vi "macro_DiffDrv_Sim_Execute.vi"() -> ()   [LabVIEW 2019, in "Trajectory_Library.lvlib"]
uses:
  Trajectory_Library.lvlib
  Enum/DCMOTOR_TYPES_ENUM.ctl
  Enum/DIFF_DRIVE_ToughBoxMini_GearChoice_ENUM.ctl
  Enum/DIFF_DRIVE_TRAIN_SIM_STATE_ENUM.ctl
  BatterySim_CalculateLoadedBatteryVoltage.vi
panel:
  in  "Right Motor Dmd (CO)":dbl
  in  "Left Motor Dmd (CO)":dbl
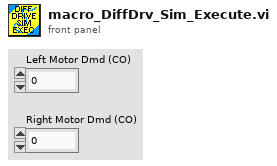
[diagram p1: front panel]
types:
  T1 = typedef "Trajectory_Library.lvlib/DIFF_DRIVE_TRAIN_SIM_STATE_ENUM.ctl" = enum16{"X_POS", "Y_POS", "HEADING", "LEFT_VEL", "RIGHT_VEL", "LEFT_DIST", "RIGHT_DIST"}
  T2 = typedef "Trajectory_Library.lvlib/DIFF_DRIVE_ToughBoxMini_GearChoice_ENUM.ctl" = enum16{"Ratio_12_75", "Ratio_10_71", "Ratio_8_45", "Ratio_7_31", "Ratio_5_95"}
  T3 = typedef "Trajectory_Library.lvlib/DCMOTOR_TYPES_ENUM.ctl" = enum16{"CIM", "AndyMark 9015", "Andy Mark RS 775 125", "Bag", "BaneBots RS 550", "BaneBots RS 775", "Falcon 500", "Mini CIM", "NEO", "NEO 550", "Romi BuiltIn", "Vex 775 Pro", "Snow Blower AM 2235A", "Bosch Seat AM 3493"}
  T4 = typedef "Trajectory_Library.lvlib/DIFF_DRIVE_SIM_SIMULATION_PARAMS.ctl" = cluster{"X Pos Meas Std Dev M":dbl, "Y Pos Meas Std Dev M":dbl, "Heading Meas Std Dev Rad":dbl, "Left Vel Meas Std Dev M/S":dbl, "Right Vel Meas Std Dev M/S":dbl, "Left Pos Meas Std Dev M":dbl, "Right Pos Meas Std Dev M":dbl}
  T5 = typedef "Trajectory_Library.lvlib/DIFF_DRIVE_SIM_MODEL_PARAMS.CTL" = cluster{"TracWidth_M":dbl, "WheelRadius_M":dbl, "Gearing":dbl, "Mass kg":dbl, "MOI kgm2":dbl, "DCMOTOR_TYPES":T3, "Num Motors":i32}
  T6 = typedef "Trajectory_Library.lvlib/DIFF_DRIVE_TRAIN_SIM.ctl" = cluster{"m_Plant":T7, "m_X":T8, "m_Y":T8, "m_U":T8, "MeasureStdDev":T8, "m_Motor":T9, "m_OriginalGearing":dbl, "m_CurrentGearing":dbl, "m_WheelRadius_M":dbl, "m_RB":dbl}
  T7 = typedef "Trajectory_Library.lvlib/LINEAR_SYSTEM.ctl" = cluster{"m_A":T8, "m_B":T8, "m_C":T8, "m_D":T8, "States":i32, "Inputs":i32, "Outputs":i32}
  T8 = typedef "NI_Matrix.lvlib/RealMatrix.ctl" = dbl[][]
  T9 = typedef "Trajectory_Library.lvlib/DCMOTOR.CTL" = cluster{"nominalVoltage_Volts":dbl, "StallTorque_NM":dbl, "StallCurrent_Amps":dbl, "FreeCurrent_Amps":dbl, "FreeSpeed_RadPerSec":dbl, "R_Ohms":dbl, "KvINV_RadPerSecPerVolt":dbl, "Kt_NMPerAmp":dbl, "L_H":dbl, "Jr_KgM2":dbl}
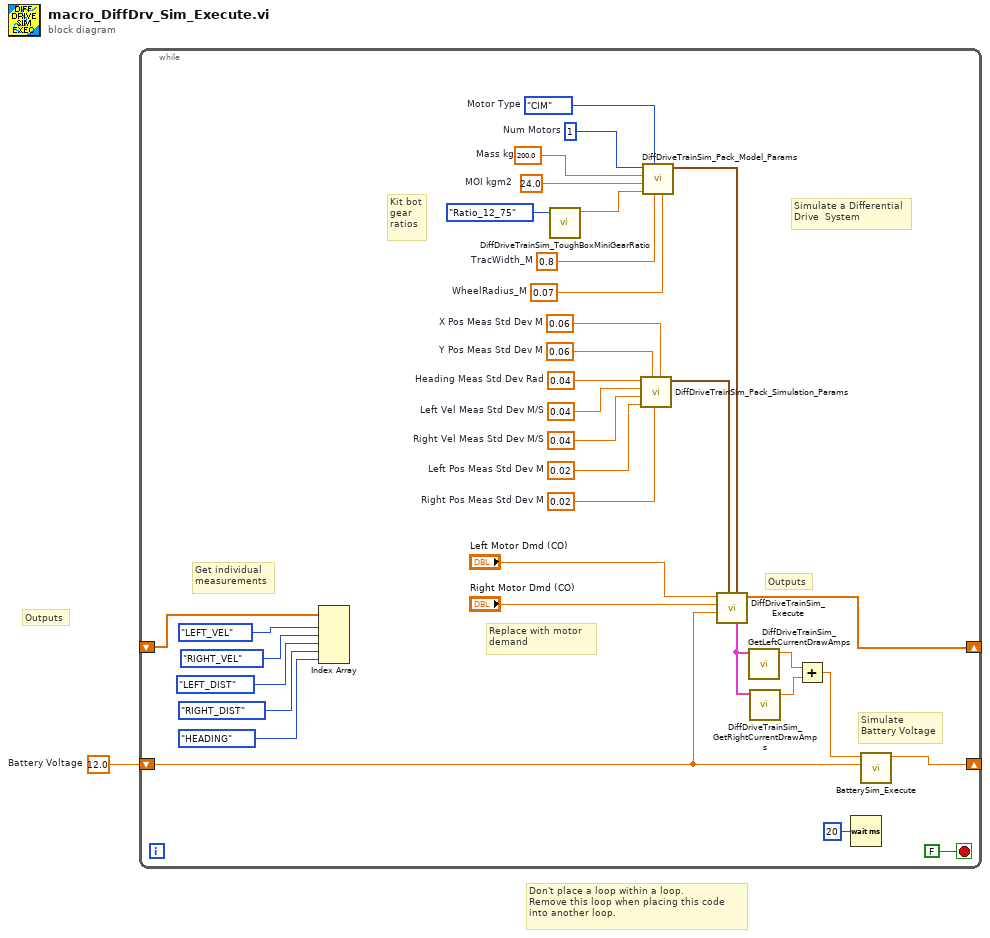
[diagram p0: block diagram]
diagram:
  w1 = 12.0  # Battery Voltage
  # "Don't place a loop within a loop. \nRemove this loop when placing this code\ninto another loop."
  # "Outputs"
  n1 = while {
    shift-right: [w31] -> _
    shift-left: w1 -> [w26]
    shift-right: [w30] -> _
    shift-left: _ -> [w7]
    stop <- FALSE stop-if-true
    w14 = 200.0  # Mass kg
    w15 = 24.0  # MOI kgm2
    w16 = 0.8  # TracWidth_M
    w17 = 0.07  # WheelRadius_M
    w18 = 0.04  # Heading Meas Std Dev Rad
    w19 = 0.04  # Left Vel Meas Std Dev M/S
    w20 = 0.04  # Right Vel Meas Std Dev M/S
    w21 = 0.02  # Left Pos Meas Std Dev M
    w22 = 0.06  # Y Pos Meas Std Dev M
    w23 = 0.02  # Right Pos Meas Std Dev M
    w24 = 0.06  # X Pos Meas Std Dev M
    w34 = 1  # Num Motors
    w35 = DCMOTOR_TYPES_ENUM."CIM"  # Motor Type
    # "Get individual\nmeasurements"
    # "Kit bot\ngear \nratios"
    # "Outputs"
    # "Replace with motor \ndemand"
    # "Simulate\nBattery Voltage"
    # "Simulate a Differential\nDrive  System"
    n2 = Index Array(array=w7, index #1=DIFF_DRIVE_TRAIN_SIM_STATE_ENUM."LEFT_VEL" ("DIFF_DRIVE_TRAIN_SIM_STATE"), index #2=DIFF_DRIVE_TRAIN_SIM_STATE_ENUM."RIGHT_VEL" ("DIFF_DRIVE_TRAIN_SIM_STATE"), index #3=DIFF_DRIVE_TRAIN_SIM_STATE_ENUM."LEFT_DIST" ("DIFF_DRIVE_TRAIN_SIM_STATE"), index #4=DIFF_DRIVE_TRAIN_SIM_STATE_ENUM."RIGHT_DIST" ("DIFF_DRIVE_TRAIN_SIM_STATE"), index #5=DIFF_DRIVE_TRAIN_SIM_STATE_ENUM."HEADING" ("DIFF_DRIVE_TRAIN_SIM_STATE")) -> ()  [unwired: 5 out]
    n3 = call "DiffDriveTrainSim_ToughBoxMiniGearRatio.vi"("ToughBoxMiniGear"=DIFF_DRIVE_ToughBoxMini_GearChoice_ENUM."Ratio_12_75") -> ("GearRatio"=w12:dbl)  [unwired: 10 in]
    n4 = call "DiffDriveTrainSim_Pack_Simulation_Params.vi"("X Pos Meas Std Dev M"=w24, "Right Pos Meas Std Dev M"=w23, "Y Pos Meas Std Dev M"=w22, "Left Pos Meas Std Dev M"=w21, "Right Vel Meas Std Dev M/S"=w20, "Left Vel Meas Std Dev M/S"=w19, "Heading Meas Std Dev Rad"=w18) -> ("DiffDriveSim_Simulation _Params"=w27:T4)  [unwired: 4 in]
    n5 = call "DiffDriveTrainSim_Pack_Model_Params.vi"("WheelRadius_M"=w17, "TracWidth_M"=w16, "DCMOTOR_TYPES"=w35, "Gearing"=w12, "MOI kgm2"=w15, "Mass kg"=w14, "Num Motors"=w34) -> ("DiffDriveSim_Model _Params"=w29:T5)  [unwired: 4 in]
    n6 = call "DiffDriveTrainSim_Execute.vi"("LinearSystem_ID_DiffDrv_Model"=w29, "ElevatorSim_Simulation _Params"=w27, "BatteryVoltage"=w26, "Right Motor Dmd"="Right Motor Dmd (CO)", "Left Motor Dmd"="Left Motor Dmd (CO)") -> ("Outputs"=w30:dbl[], "out DiffDriveTrainSim"=w11:T6)  [unwired: 4 in, 1 out]
    n7 = call "DiffDriveTrainSim_GetLeftCurrentDrawAmps.vi"("DiffDriveTrainSim"=w11) -> ("LeftCurrentDraw_Amps"=w10:dbl)  [unwired: 10 in]
    n8 = call "DiffDriveTrainSim_GetRightCurrentDrawAmps.vi"("DiffDriveTrainSim"=w11) -> ("RightCurrentDraw_Amps"=w9:dbl)  [unwired: 10 in]
    n9 = Add(x=w10, y=w9) -> (x+y=w8:dbl)
    n10 = Wait (ms)(milliseconds to wait=u32 20) -> ()  [unwired: 1 out]
    n11 = call "BatterySim_Execute.vi"("Nominal Battery Voltage"=w26, "Current"=w8) -> ("Voltage"=w31:dbl)  [unwired: 9 in]
  }
